vi "Main.vi"() -> ()   [LabVIEW 2019]
doc: "The myRIO Project template acquires acceleration data from the onboard accelerometer and displays the changes of acceleration values in a waveform chart."
uses:
  <vilib>/Platform/TimedLoop/XDataNode/timing_clust.ctl
  <vilib>/Platform/TimedLoop/XDataNode/nitl_modes.ctl
  <vilib>/Platform/TimedLoop/XDataNode/wakeup.ctl
  <vilib>/myRIO/Instrument Drivers/Onboard IO/AI/typedefs/AI Reference.ctl
  <vilib>/myRIO/Common/Instrument Driver Framework/Utilities/typedefs/myRIO Generic Hardware Reference.ctl
  <vilib>/myRIO/Common/Instrument Driver Framework/Utilities/typedefs/Hardware Version Enum.ctl
  <vilib>/myRIO/Common/Instrument Driver Framework/Utilities/typedefs/myRIO v1.0 Reference.ctl
  <vilib>/myRIO/Common/Instrument Driver Framework/Utilities/typedefs/Generic FPGA Reference.ctl
  <vilib>/myRIO/Common/Instrument Driver Framework/myRIO v1.0/AI/typedefs/AI Channels List.ctl
  <vilib>/myRIO/Common/Instrument Driver Framework/myRIO v1.0/AI/typedefs/AI Channels Enum.ctl
  <vilib>/myRIO/Common/Instrument Driver Framework/Utilities/typedefs/Analog Scaling Constants List.ctl
  <vilib>/myRIO/Common/Instrument Driver Framework/Utilities/typedefs/Analog Scaling Constants.ctl
  <vilib>/userdefined/High Color/nirio_resource_hc.ctl
  <vilib>/myRIO/Instrument Drivers/Onboard IO/DIO/typedefs/DIO Reference.ctl
  <vilib>/myRIO/Common/Instrument Driver Framework/myRIO v1.0/DIO/typedefs/DIO Channels List.ctl
  <vilib>/myRIO/Common/Instrument Driver Framework/myRIO v1.0/DIO/typedefs/DIO Channels Enum.ctl
  <vilib>/myRIO/Common/Instrument Driver Framework/myRIO v1.0/Encoder/typedefs/Encoder Signal Mode.ctl
  <vilib>/myRIO/Instrument Drivers/Onboard IO/Encoder/typedefs/Encoder Reference.ctl
  <vilib>/myRIO/Common/Instrument Driver Framework/myRIO v1.0/Encoder/typedefs/Encoder Channels Enum.ctl
  <vilib>/myRIO/Common/Instrument Driver Framework/myRIO v1.0/Encoder/typedefs/Encoder Configuration v1.0.ctl
  <vilib>/myRIO/Instrument Drivers/Onboard IO/AO/typedefs/AO Reference.ctl
  <vilib>/myRIO/Common/Instrument Driver Framework/myRIO v1.0/AO/typedefs/AO Channels List.ctl
  <vilib>/myRIO/Common/Instrument Driver Framework/myRIO v1.0/AO/typedefs/AO Channels Enum.ctl
  <vilib>/myRIO/Common/Instrument Driver Framework/Utilities/vis/Is FPGA Ref Available.vi
  <vilib>/myRIO/Common/Instrument Driver Framework/myRIO v1.0/AI/vis/myRIO v1.1 Open AI.vi
  <vilib>/myRIO/Instrument Drivers/Onboard IO/AI/vis/Read.vi
  <vilib>/myRIO/Common/Instrument Driver Framework/myRIO v1.0/DIO/vis/myRIO v1.1 Open DIO.vi
  <vilib>/myRIO/Instrument Drivers/Onboard IO/DIO/vis/Read.vi
  <vilib>/myRIO/Common/Instrument Driver Framework/myRIO v1.0/Encoder/vis/myRIO v1.1 Open Encoder.vi
  <vilib>/myRIO/Instrument Drivers/Onboard IO/Encoder/vis/Read.vi
  <vilib>/myRIO/Common/Instrument Driver Framework/myRIO v1.0/AO/vis/myRIO v1.1 Open AO.vi
  <vilib>/myRIO/Instrument Drivers/Onboard IO/AO/vis/Write.vi
  <vilib>/myRIO/Common/Instrument Driver Framework/Utilities/vis/Validate Channels.vi
  <vilib>/myRIO/Common/Instrument Driver Framework/myRIO v1.0/AI/vis/myRIO v1.0 Reserve AI.vi
  <vilib>/myRIO/Common/Instrument Driver Framework/myRIO v1.0/DIO/vis/myRIO v1.0 Reserve DIO.vi
  <vilib>/myRIO/Common/Instrument Driver Framework/myRIO v1.0/Encoder/vis/myRIO v1.0 Reserve Encoder.vi
  <vilib>/myRIO/Common/Instrument Driver Framework/myRIO v1.0/AO/vis/myRIO v1.0 Reserve AO.vi
  <vilib>/myRIO/Common/Instrument Driver Framework/myRIO v1.0/AI/vis/myRIO v1.0 Build MUX Configuration AI.vi
  <vilib>/myRIO/Common/Instrument Driver Framework/myRIO v1.0/Resource Manager/vis/myRIO v1.0 Reserve Channel List.vi
  <vilib>/myRIO/Common/Instrument Driver Framework/myRIO v1.0/DIO/vis/myRIO v1.0 Build MUX Configuration DIO.vi
  <vilib>/myRIO/Common/Instrument Driver Framework/myRIO v1.0/Encoder/vis/myRIO v1.0 Build MUX Configuration Encoder.vi
  <vilib>/myRIO/Common/Instrument Driver Framework/myRIO v1.0/AO/vis/myRIO v1.0 Build MUX Configuration AO.vi
  <vilib>/myRIO/Common/Instrument Driver Framework/myRIO v1.0/Resource Manager/vis/myRIO v1.0 Reserve Channel.vi
  <vilib>/myRIO/Common/Instrument Driver Framework/myRIO v1.0/Resource Manager/vis/myRIO v1.0 Unreserve Channel.vi
  <vilib>/myRIO/Common/Instrument Driver Framework/myRIO v1.0/Resource Manager/vis/myRIO v1.0 Create Configuration List.vi
  <vilib>/myRIO/Common/Instrument Driver Framework/myRIO v1.0/Resource Manager/vis/myRIO v1.0 Build Mutex Name.vi
  <vilib>/Utility/VariantDataType/GetNumericInfo.vi
  <vilib>/Utility/error.llb/Error Cluster From Error Code.vi
  <vilib>/myRIO/Common/Instrument Driver Framework/myRIO v1.0/myRIO v1.1 Open.vi
  <vilib>/myRIO/Common/Instrument Driver Framework/myRIO v1.0/AI/vis/myRIO v1.0 Get Scaling Constants AI.vi
  <vilib>/myRIO/Common/Instrument Driver Framework/Utilities/vis/IO Manager.vi
  <vilib>/myRIO/Common/Instrument Driver Framework/Utilities/vis/Configuration Manager.vi
  <vilib>/myRIO/Common/Instrument Driver Framework/myRIO v1.0/myRIO v1.0 Close.vi
  <vilib>/myRIO/Common/Instrument Driver Framework/myRIO v1.0/AI/vis/myRIO v1.0 Read AI.vi
  <vilib>/myRIO/Common/Instrument Driver Framework/myRIO v1.0/Resource Manager/vis/myRIO v1.0 Configure IO.vi
  <vilib>/myRIO/Common/Instrument Driver Framework/myRIO v1.0/DIO/vis/myRIO v1.0 Read DIO.vi
  <vilib>/myRIO/Common/Instrument Driver Framework/myRIO v1.0/Encoder/vis/myRIO v1.0 Configure Encoder.vi
  <vilib>/myRIO/Common/Instrument Driver Framework/myRIO v1.0/Encoder/vis/myRIO v1.0 Read Encoder.vi
  <vilib>/myRIO/Common/Instrument Driver Framework/myRIO v1.0/AO/vis/myRIO v1.0 Get Scaling Constants AO.vi
  <vilib>/myRIO/Common/Instrument Driver Framework/myRIO v1.0/AO/vis/myRIO v1.0 Write AO.vi
  <vilib>/Platform/TimedLoop/XDataNode/XDataNode.xnode
  <vilib>/myRIO/Express VI/Onboard IO/AI/AI Express VI.xnode
  <vilib>/myRIO/Instrument Drivers/Onboard IO/AI/vis/myRIO AI Open.xnode
  <vilib>/myRIO/Express VI/Onboard IO/DI/DI Express VI.xnode
  <vilib>/myRIO/Instrument Drivers/Onboard IO/DIO/vis/myRIO DIO Open.xnode
  <vilib>/myRIO/Express VI/Onboard IO/Encoder/Encoder Express VI.xnode
  <vilib>/myRIO/Instrument Drivers/Onboard IO/Encoder/vis/myRIO Encoder Open.xnode
  <vilib>/myRIO/Common/Instrument Driver Framework/myRIO v1.0/Encoder/typedefs/Encoder Count Direction Enum.ctl
  <vilib>/myRIO/Express VI/Onboard IO/AO/AO Express VI.xnode
  <vilib>/myRIO/Instrument Drivers/Onboard IO/AO/vis/myRIO AO Open.xnode
  <vilib>/Platform/TimedLoop/XDataNode/XDNodeRunTimeDep.lvlib
  <vilib>/myRIO/Instrument Drivers/Onboard IO/AO/AO.lvlib
  <vilib>/ptbypt/NI_PtbyPt.lvlib
  <vilib>/myRIO/Instrument Drivers/Onboard IO/DIO/DIO.lvlib
  <vilib>/myRIO/Instrument Drivers/Onboard IO/AI/AI.lvlib
  <vilib>/myRIO/Instrument Drivers/Onboard IO/Encoder/Encoder.lvlib
panel:
  in  "Period":i64=1000
  out "Setpoint":dbl
  out "Kp":dbl
  out "Kd":dbl
  out "Ki":dbl
  in  "Output Gain":dbl=1.0
  in  "Output Range":cluster{"output high":dbl, "output low":dbl}={"output high"=100.0, "output low"=-100.0} {"output low" format="%.2f"; "output high" format="%.2f"}
  in  "Stop Button":bool
  out "Response Graph":cluster{dbl, "sine wave":dbl}(graph)
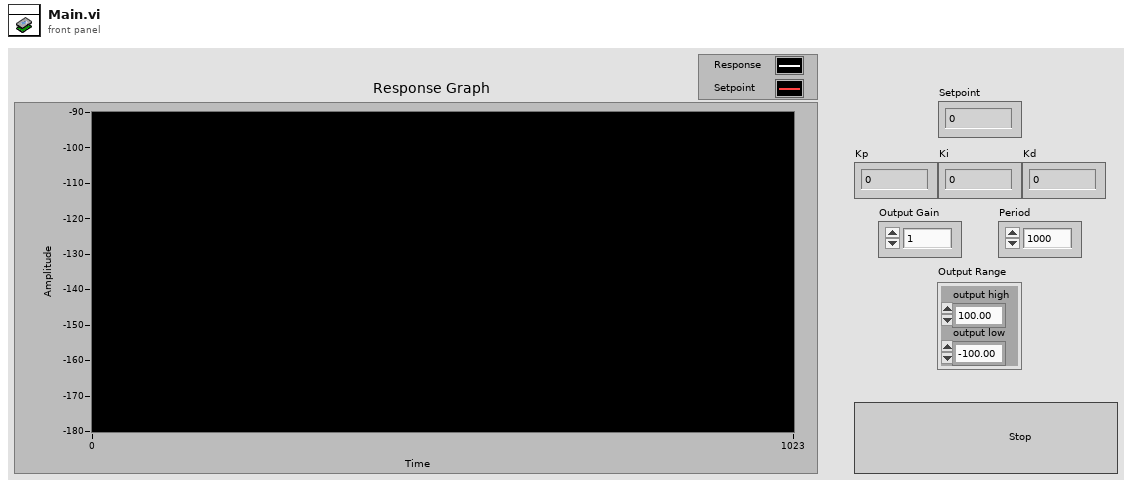
[diagram p1: front panel]
types:
  T1 = typedef "XDNodeRunTimeDep.lvlib/timing_clust.ctl" = cluster{"Expected End [f-1]":u64, "Actual End [f-1]":u64, "Finished Late? [f-1]":bool, "Expected End [i-1]":u64, "Actual End [i-1]":u64, "Finished Late? [i-1]":bool, "Expected Start [i]":u64, "Actual Start [i]":u64, "Expected Start [f]":u64, "Actual Start [f]":u64, "Source Name":string, "Structure Name":string, "Period":i64, "Deadline":i64, "Offset":i64, "Start":i64, "Priority":i32, "Timeout":i32, "Mode":T2, "Wakeup Reason":T3, "Error":errorcluster, "Source Type":string, "Secondary Source Type":string, "Global End Time":u64, "Global Start Time":u64, "Frame Duration":u64, "Iteration Duration":u64, "Assigned CPU":i32, "I/O Scan Engine Mode":u32}
  T2 = typedef "XDNodeRunTimeDep.lvlib/nitl_modes.ctl" = enum32{"No Change", "Process missed periods, maintain original phase", "Discard missed periods, maintain original phase", "Process missed periods, ignore original phase", "Discard missed periods, ignore original phase"}
  T3 = typedef "XDNodeRunTimeDep.lvlib/wakeup.ctl" = enum32{"Normal", "Aborted", "Asynchronous wakeup", "Timing source error", "Timed loop error", "Timeout"}
  T4 = typedef "DIO.lvlib/DIO Reference.ctl" = cluster{"myRIO Reference":T5, "DIO Channels List":T9}
  T5 = typedef "myRIO Generic Hardware Reference.ctl" = cluster{"myRIO Model":T6, "myRIO Hardware Reference":T7}
  T6 = typedef "Hardware Version Enum.ctl" = enum16{"Unknown", "myRIO-1900", "myRIO-1950", "roboRIO", "NI ELVIS RIO CM", "ELVIS III"}
  T7 = typedef "myRIO v1.0 Reference.ctl" = cluster{"Generic FPGA Reference":T8, "Allow multiple opens":bool}
  T8 = typedef "Generic FPGA Reference.ctl" = refnum<k20>
  T9 = typedef "DIO Channels List.ctl" = T10[]
  T10 = typedef "DIO Channels Enum.ctl" = enum16{"Not Connected", "C/DIO0", "C/DIO1", "C/DIO2", "C/DIO3", "C/DIO4", "C/DIO5", "C/DIO6", "C/DIO7", "A/DIO0", "A/DIO1", "A/DIO2", "A/DIO3", "A/DIO4", "A/DIO5", "A/DIO6", "A/DIO7", "A/DIO8", "A/DIO9", "A/DIO10", "A/DIO11", "A/DIO12", "A/DIO13", "A/DIO14", "A/DIO15", "A/DIO16", "A/DIO17", "A/DIO18", "A/DIO19", "B/DIO0", "B/DIO1", "B/DIO2", "B/DIO3", "B/DIO4", "B/DIO5", "B/DIO6", "B/DIO7", "B/DIO8", "B/DIO9", "B/DIO10", "B/DIO11", "B/DIO12", "B/DIO13", "B/DIO14", "B/DIO15", "B/DIO16", "B/DIO17", "B/DIO18", "B/DIO19", "LED0", "LED1", "LED2", "LED3", "Button0", "DIO/DIO0", "DIO/DIO1", "DIO/DIO2", "DIO/DIO3", "DIO/DIO4", "DIO/DIO5", "DIO/DIO6", "DIO/DIO7", "DIO/DIO8", "DIO/DIO9", "SPI/CS0", "SPI/CS1", "SPI/CS2", "SPI/CS3", "LED RADIO (Green)", "LED RADIO (Red)", "LED COMM (Green)", "LED COMM (Red)", "LED MODE (Green)", "LED MODE (Red)"}
  T11 = typedef "nirio_resource_hc.ctl" = tag
  T12 = typedef "AI.lvlib/AI Reference.ctl" = cluster{"myRIO Reference":T5, "AI Channels List":T13, "AI Scaling Constants List":T15}
  T13 = typedef "AI Channels List.ctl" = T14[]
  T14 = typedef "AI Channels Enum.ctl" = enum16{"Not Connected", "AudioIn/Left", "AudioIn/Right", "C/AI0", "C/AI1", "A/AI0", "A/AI1", "A/AI2", "A/AI3", "A/AI4", "A/AI5", "A/AI6", "A/AI7", "B/AI0", "B/AI1", "B/AI2", "B/AI3", "B/AI4", "B/AI5", "B/AI6", "B/AI7", "AI/AI0", "AI/AI1", "AI/AI2", "AI/AI3", "A/AI0 (DIFF)", "A/AI1 (DIFF)", "A/AI2 (DIFF)", "A/AI3 (DIFF)", "B/AI0 (DIFF)", "B/AI1 (DIFF)", "B/AI2 (DIFF)", "B/AI3 (DIFF)"}
  T15 = typedef "Analog Scaling Constants List.ctl" = T16[]
  T16 = typedef "Analog Scaling Constants.ctl" = cluster{"LSB Weight (Volts)":dbl, "Offset (Volts)":dbl, "Signed?":bool}
  T17 = typedef "AO.lvlib/AO Reference.ctl" = cluster{"myRIO Reference":T5, "AO Channel List":T18, "AO Scaling Constant List":T15}
  T18 = typedef "AO Channels List.ctl" = T19[]
  T19 = typedef "AO Channels Enum.ctl" = enum16{"Not Connected", "AudioOut/Left", "AudioOut/Right", "C/AO0", "C/AO1", "A/AO0", "A/AO1", "B/AO0", "B/AO1"}
  T20 = typedef "Encoder.lvlib/Encoder Reference.ctl" = cluster{"myRIO Reference":T5, "Encoder Channels Enum":T21}
  T21 = typedef "Encoder Channels Enum.ctl" = enum16{"Not Connected", "C/ENC0", "C/ENC1", "A/ENC", "A/ENC0", "A/ENC1", "A/ENC2", "A/ENC3", "A/ENC4", "A/ENC5", "A/ENC6", "A/ENC7", "A/ENC8", "A/ENC9", "B/ENC", "B/ENC0", "B/ENC1", "B/ENC2", "B/ENC3", "B/ENC4", "B/ENC5", "B/ENC6", "B/ENC7", "B/ENC8", "B/ENC9", "DIO/ENC0", "DIO/ENC1", "DIO/ENC2", "DIO/ENC3", "DIO/ENC4"}
  T22 = typedef "Encoder Signal Mode.ctl" = enum16{"Quadrature phase signal", "Step and direction signal"}
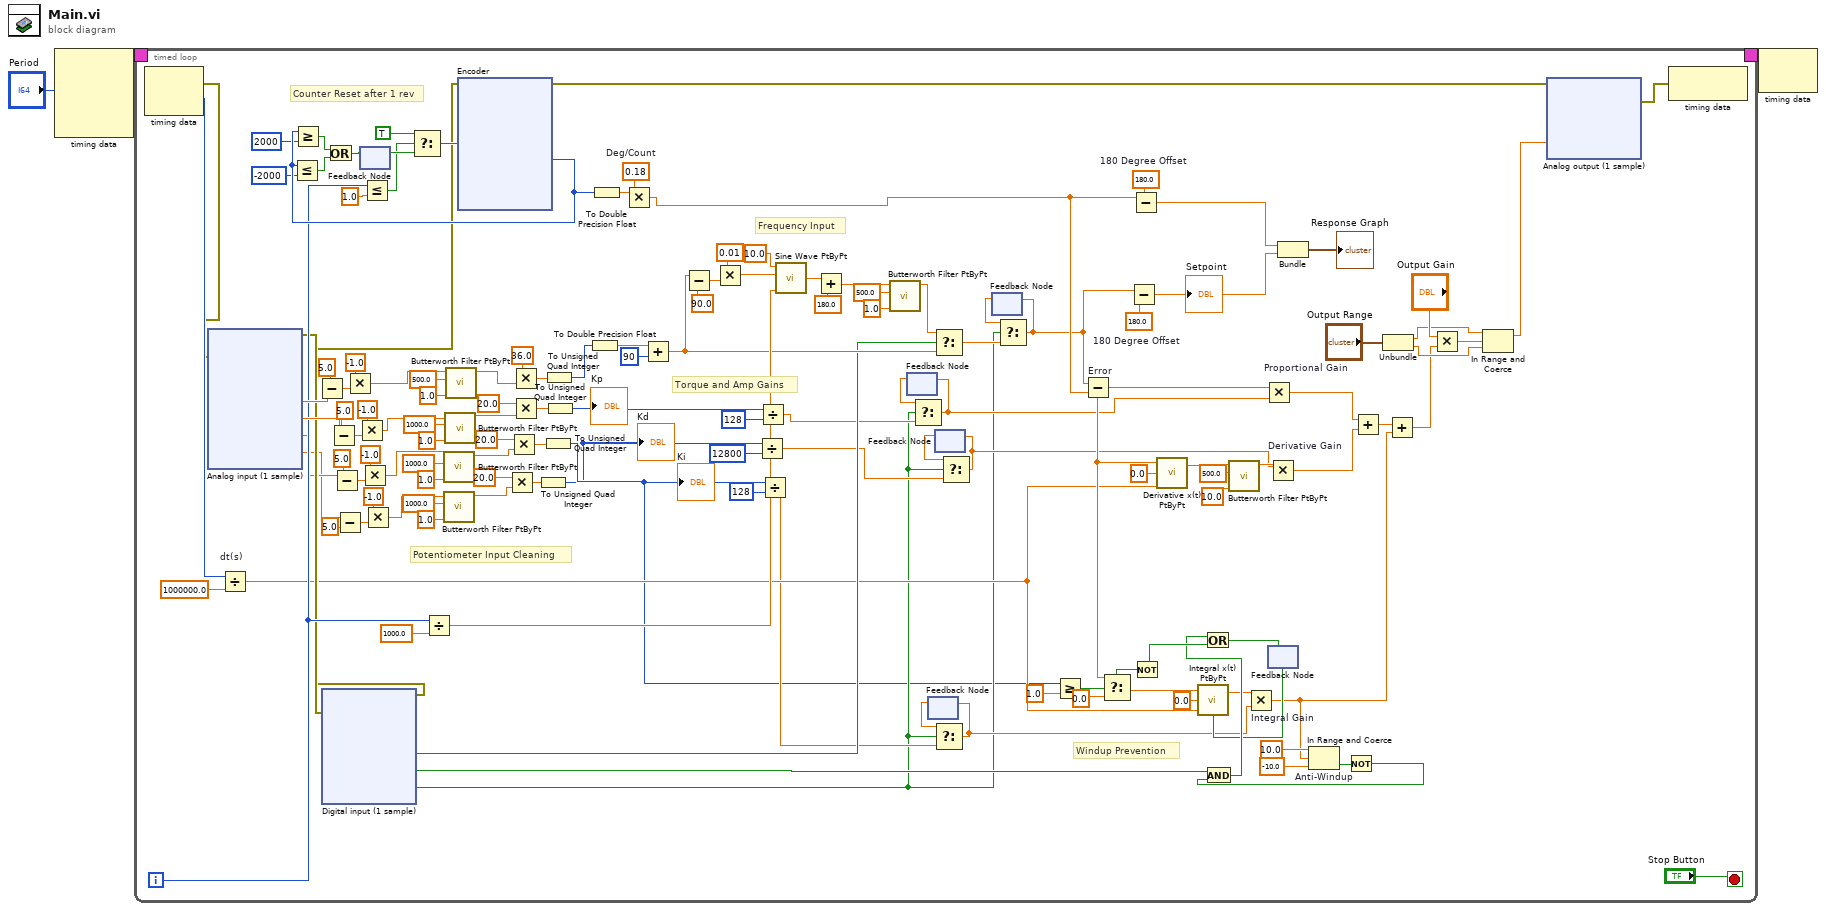
[diagram p0: block diagram]
diagram:
  n1 = node-c288("Period") -> (w3:T1)  [unwired: 3 in]
  n2 = timed-loop {
    timing: w3 -> [_]
    timing-out: [_] -> w2
    i -> [w59]
    stop <- "Stop Button" stop-if-true
    w51 = 180.0  # 180 Degree Offset
    w127 = 180.0  # 180 Degree Offset
    w140 = 0.18  # Deg/Count
    # "Counter Reset after 1 rev"
    # "Windup Prevention"
    # "Torque and Amp Gains"
    # "Potentiometer Input Cleaning"
    # "Frequency Input"
    n3 = node-c288() -> (w35:errorcluster, w67:i64)  [unwired: 1 in]
    n4 = xnode "Analog input (1 sample)"("error in (no error)"=w35) -> ("Setpont (A/AI0 (Pin 3))"=w91:dbl, "Proportional (A/AI1 (Pin 5))"=w83:dbl, "Derivative (A/AI2 (Pin 7))"=w29:dbl, "Integral (A/AI3 (Pin 9))"=w28:dbl, "error out"=w34:errorcluster)
    n5 = Divide "dt(s)"(x=w67, y=1000000.0) -> (x/y=w31:dbl)
    n6 = Subtract(x=w91, y=5.0) -> (x-y=w89:dbl)
    n7 = xnode "Digital input (1 sample)"("error in (no error)"=w34) -> ("Frequency Input (C/DIO0 (DIO0))"=w46:bool, "Anti-Windup (C/DIO1 (DIO1))"=w39:bool, "Hold (C/DIO2 (DIO2))"=w6:bool, "error out"=w33:errorcluster)
    n8 = Subtract(x=w83, y=5.0) -> (x-y=w85:dbl)
    n9 = Subtract(x=w29, y=5.0) -> (x-y=w80:dbl)
    n10 = Subtract(x=w28, y=5.0) -> (x-y=w76:dbl)
    n11 = Multiply(x=-1.0, y=w89) -> (x*y=w87:dbl)
    n12 = Multiply(x=-1.0, y=w85) -> (x*y=w82:dbl)
    n13 = feedback #1() -> (w133:bool)  [unwired: 1 in]
    n14 = Multiply(x=-1.0, y=w80) -> (x*y=w78:dbl)
    n15 = Less Or Equal?(x=w59, y=1.0) -> (x <= y?=w131:bool)
    n16 = Multiply(x=-1.0, y=w76) -> (x*y=w74:dbl)
    n17 = Select(t=TRUE, s=w131, f=w133) -> (s? t:f=w129:bool)
    n18 = Divide(x=w59, y=1000.0) -> (x/y=w58:dbl)
    n19 = call <vilib>:"Butterworth Filter PtByPt.vi"("low cutoff freq: fl"=1.0, "sampling freq: fs"=1000.0, "x"=w78) -> ("Filtered x"=w98:dbl)  [unwired: 6 in, 1 out]
    n20 = call <vilib>:"Butterworth Filter PtByPt.vi"("low cutoff freq: fl"=1.0, "sampling freq: fs"=1000.0, "x"=w74) -> ("Filtered x"=w96:dbl)  [unwired: 6 in, 1 out]
    n21 = call <vilib>:"Butterworth Filter PtByPt.vi"("low cutoff freq: fl"=1.0, "sampling freq: fs"=1000.0, "x"=w82) -> ("Filtered x"=w101:dbl)  [unwired: 6 in, 1 out]
    n22 = call <vilib>:"Butterworth Filter PtByPt.vi"("low cutoff freq: fl"=1.0, "sampling freq: fs"=500.0, "x"=w87) -> ("Filtered x"=w107:dbl)  [unwired: 6 in, 1 out]
    n23 = xnode "Encoder"("Reset Counter"=w129, "error in (no error)"=w33) -> ("Counter Value"=w137:i32, "error out"=w32:errorcluster)  [unwired: 2 out]
    n24 = Less Or Equal?(x=w137, y=-2000) -> (x <= y?=w138:bool)
    n25 = Greater Or Equal?(x=w137, y=2000) -> (x >= y?=w139:bool)
    n26 = Or(x=w139, y=w138) -> (x .or. y?=w134:bool)
    n27 = feedback-in #1(w134) -> ()
    n28 = Multiply(x=20.0, y=w96) -> (x*y=w93:dbl)
    n29 = Multiply(x=20.0, y=w98) -> (x*y=w94:dbl)
    n30 = Multiply(x=36.0, y=w107) -> (x*y=w92:dbl)
    n31 = Multiply(x=20.0, y=w101) -> (x*y=w95:dbl)
    n32 = To Unsigned Quad Integer(1:w93) -> (0:w4:u64)
    "Kd" <- w4
    n33 = To Unsigned Quad Integer(1:w94) -> (0:w5:u64)
    "Ki" <- w5
    n34 = To Unsigned Quad Integer(1:w92) -> (0:w70:u64)
    n35 = To Unsigned Quad Integer(1:w95) -> (0:w73:u64)
    "Kp" <- w73
    n36 = To Double Precision Float(number=w70) -> (double precision float=w68:dbl)
    n37 = To Double Precision Float(number=w137) -> (double precision float=w141:dbl)
    n38 = Multiply(x=w141, y=w140) -> (x*y=w19:dbl)
    n39 = Add(x=w68, y=u64 90) -> (x+y=w57:dbl)
    n40 = Subtract(x=w57, y=90.0) -> (x-y=w55:dbl)
    n41 = Multiply(x=0.01, y=w55) -> (x*y=w53:dbl)
    n42 = Divide(x=w4, y=u64 12800) -> (x/y=w11:dbl)
    n43 = Divide(x=w73, y=u64 128) -> (x/y=w14:dbl)
    n44 = Divide(x=w5, y=u64 128) -> (x/y=w8:dbl)
    n45 = call <vilib>:"Sine Wave PtByPt.vi"("time"=w58, "frequency"=w53, "amplitude"=10.0) -> ("sine wave"=w50:dbl)  [unwired: 1 in]
    n46 = Add(x=w50, y=180.0) -> (x+y=w23:dbl)
    n47 = call <vilib>:"Butterworth Filter PtByPt.vi"("low cutoff freq: fl"=1.0, "sampling freq: fs"=500.0, "x"=w23) -> ("Filtered x"=w22:dbl)  [unwired: 6 in, 1 out]
    n48 = feedback #2() -> (w15:dbl)  [unwired: 1 in]
    n49 = Select(t=w15, s=w6, f=w14) -> (s? t:f=w13:dbl)
    n50 = feedback-in #2(w13) -> ()
    n51 = feedback #3() -> (w9:dbl)  [unwired: 1 in]
    n52 = Select(t=w22, s=w46, f=w57) -> (s? t:f=w18:dbl)
    n53 = Select(t=w9, s=w6, f=w8) -> (s? t:f=w7:dbl)
    n54 = feedback-in #3(w7) -> ()
    n55 = feedback #4() -> (w12:dbl)  [unwired: 1 in]
    n56 = Select(t=w12, s=w6, f=w11) -> (s? t:f=w10:dbl)
    n57 = feedback-in #4(w10) -> ()
    n58 = feedback #5() -> (w16:dbl)  [unwired: 1 in]
    n59 = Select(t=w16, s=w6, f=w18) -> (s? t:f=w17:dbl)
    n60 = feedback-in #5(w17) -> ()
    n61 = Greater Or Equal?(x=w5, y=1.0) -> (x >= y?=w62:bool)
    n62 = Subtract "Error"(x=w17, y=w19) -> (x-y=w64:dbl)
    n63 = Select(t=w64, s=w62, f=0.0) -> (s? t:f=w65:dbl)
    n64 = Subtract(x=w17, y=w51) -> (x-y=w26:dbl)
    "Setpoint" <- w26
    n65 = Subtract(x=w19, y=w127) -> (x-y=w102:dbl)
    n66 = Not(x=w62) -> (.not. x?=w43:bool)
    n67 = call <vilib>:"Derivative x(t) PtByPt.vi"("dt"=w31, "initial condition"=0.0, "x"=w64) -> ("dx/dt"=w121:dbl)  [unwired: 1 in, 1 out]
    n68 = call <vilib>:"Butterworth Filter PtByPt.vi"("low cutoff freq: fl"=10.0, "sampling freq: fs"=500.0, "x"=w121) -> ("Filtered x"=w117:dbl)  [unwired: 6 in, 1 out]
    n69 = Multiply "Proportional Gain"(x=w64, y=w13) -> (x*y=w124:dbl)
    n70 = Multiply "Derivative Gain"(x=w10, y=w117) -> (x*y=w125:dbl)
    n71 = feedback #6() -> (w40:bool)  [unwired: 1 in]
    n72 = call <vilib>:"Integral x(t) PtByPt.vi"("initialize"=w40, "dt"=w31, "initial condition"=0.0, "x"=w65) -> ("integral x(t)"=w30:dbl)  [unwired: 1 out]
    n73 = Multiply "Integral Gain"(x=w30, y=w7) -> (x*y=w27:dbl)
    n74 = Bundle(w102, w26) -> (→"Response Graph":cluster{dbl, dbl})  [unwired: 1 in]
    n75 = In Range and Coerce "Anti-Windup"(upper limit=10.0, x=w27, lower limit=-10.0) -> (In Range?=w45:bool)  [unwired: 1 out]
    n76 = Not(x=w45) -> (.not. x?=w44:bool)
    n77 = And(x=w39, y=w44) -> (x .and. y?=w42:bool)
    n78 = Or(x=w42, y=w43) -> (x .or. y?=w41:bool)
    n79 = feedback-in #6(w41) -> ()
    n80 = Add(x=w124, y=w125) -> (x+y=w119:dbl)
    n81 = Unbundle("Output Range") -> ("output high"=w115:dbl, "output low"=w114:dbl)
    n82 = Add(x=w119, y=w27) -> (x+y=w66:dbl)
    n83 = Multiply(x="Output Gain", y=w66) -> (x*y=w122:dbl)
    n84 = In Range and Coerce(upper limit=w115, x=w122, lower limit=w114) -> (coerced(x)=w20:dbl)  [unwired: 1 out]
    n85 = xnode "Analog output (1 sample)"("C/AO0 (AO0)"=w20, "error in (no error)"=w32) -> ("error out"=w113:errorcluster)
    n86 = node-c288(w113) -> ()  [unwired: 1 out]
  }
  n87 = node-c288(w2) -> ()  [unwired: 1 out]
